vi "NumberConversion.vi"(1 "Numeric":dbl) -> (0 "number":i32)   [LabVIEW 2015]
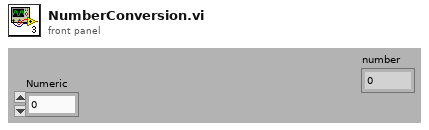
[diagram p1: front panel]
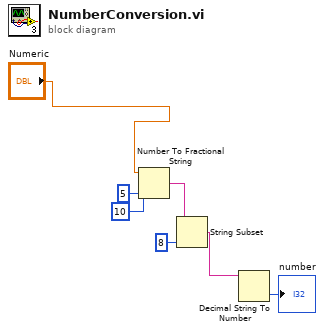
[diagram p0: block diagram]
diagram:
  n1 = Number To Fractional String(number="Numeric", width (-)=i16 10, precision (6)=i16 5) -> (F-format string=w5:string)  [unwired: 1 in]
  n2 = String Subset(string=w5, length (rest)=8 ("length (rest)")) -> (substring=w3:string)  [unwired: 1 in]
  n3 = Decimal String To Number(string=w3) -> (number=→"number":i32)  [unwired: 2 in, 1 out]
